vi "ActorDatabase-UpdateReplytoActor.vi"(8 "error in (no error)":errorcluster, 10 "Update Successful":bool, 11 "Database-Actor in":refnum<class "PartCertDatabase-Actor.lvclass">) -> (0 "error out":errorcluster, 3 "Database-Actor out":refnum<class "PartCertDatabase-Actor.lvclass">)   [LabVIEW 2013, in "PartCertDatabase-Actor.lvclass"]
uses:
  PartCertDatabase-Actor.lvclass
  ftw-dataflow/Core/src/Reflection/FTW-Reflection-Type.vi
  ftw-dataflow/Core/src/JSON/FTW-JSON-Core-LibraryFilepath.vi
  ftw-dataflow/Core/src/JSON/FTW-JSON-Core-GetFlattenedValue.vi
  ftw-dataflow/Core/src/JSON/FTW-JSON-Core-LibraryError.vi
  ftw-dataflow/Core/utils/CodeGen/JSON Deserialize/FTW-JSON-Deserialize.xnode
  PCert-Container/ERP-ConfigPageNewFeather/PCert-ConfigPageNF.lvclass
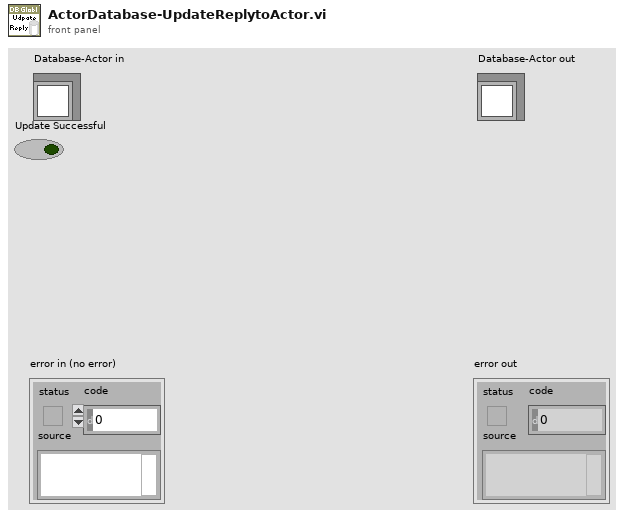
[diagram p1: front panel]
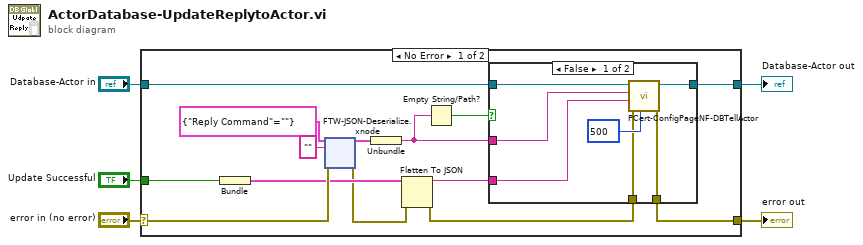
[diagram p0: block diagram]
diagram:
  n1 = case shown="No Error" "error in (no error)" {
    selector: "error in (no error)" -> [w17 w64]
    tunnel: [w16 w64] -> w4
    tunnel: [w18 w63] -> w2
    tunnel: "Database-Actor in" -> [w19 w63]
    tunnel: "Update Successful" -> [w15 _]
    frame No Error {
      n2 = Bundle("Update Successful"=w15) -> (w14:cluster{"Update Successful":bool})  [unwired: 1 in]
      n3 = xnode "FTW-JSON-Deserialize.xnode"("Type and Defaults"=cluster{"Reply Command":string} {"Reply Command"=""} ("output cluster"), "JSON String"="", "error in"=w17) -> ("Values"=w7:cluster{"Reply Command":string}, "error out"=w13:errorcluster)
      n4 = Unbundle(w7) -> ("Reply Command"=w10:string)
      n5 = Flatten To JSON(anything=w14, error in (no error)=w13) -> (JSON string=w11:string, 11:w12:errorcluster)  [unwired: 1 in]
      n6 = Empty String/Path?(string/path=w10) -> (empty?=w9:bool)
      n7 = case shown="False" w9 {
        tunnel: w19 -> [w25 w28]
        tunnel: [w24 w28] -> w18
        tunnel: [w23 w27] -> w16
        tunnel: w12 -> [w22 w27]
        tunnel: w11 -> [w21 _]
        tunnel: w10 -> [w20 _]
        frame False {
          n8 = call "PCert-ConfigPageNF-DBTellActor.vi"("Timeout"=500, "error in (no error)"=w22, "Message Body"=w21, "Message Header"=w20, "ERP-ConfigPageNF in"=w25) -> ("error out"=w23:errorcluster, "ERP-ConfigPageNF out"=w24:refnum<class "PartCertDatabase-Actor.lvclass">)  [unwired: 4 in, 1 out]
        }
        frame True {
          # "No Reply Needed"
        }
      }
    }
    frame Error {
    }
  }
  "error out" <- w4
  "Database-Actor out" <- w2
